vi "SVPWMTimingAlphaBetaFXP_src.vi"(0 "alpha":fxp<+/-,32,4> caption="voltage alpha", 1 "max":fxp<+/-,32,4>=0.999969482421875 caption="max voltage", 2 "Period":u32, 5 "beta":fxp<+/-,32,4> caption="voltage beta") -> (4 "U_Timing":T1, 6 "V_Timing":T1, 8 "W_timing":T1, 15 "Sector":u8)   [LabVIEW 2015]
uses:
  ON_OFF_timing.ctl
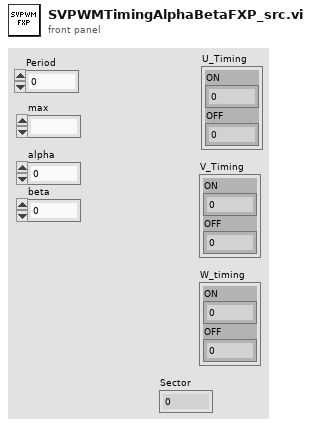
[diagram p1: front panel]
types:
  T1 = typedef "ON_OFF_timing.ctl" = cluster{"ON":u32, "OFF":u32}
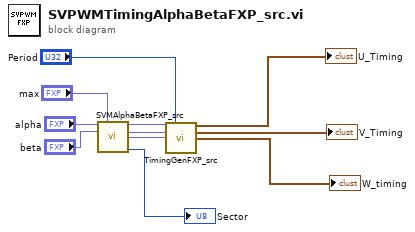
[diagram p0: block diagram]
diagram:
  n1 = call "SVMAlphaBetaFXP_src.vi"("alpha"="alpha", "max"="max", "beta"="beta") -> ("Upercent"=w11:fxp<+/-,32,4>, "Vpercent"=w10:fxp<+/-,32,4>, "Wpercent"=w9:fxp<+/-,32,4>, "Sector"=→"Sector":u8)  [unwired: 9 in]
  n2 = call "TimingGenFXP_src.vi"("Upercent"=w11, "Period"="Period", "Vpercent"=w10, "Wpercent"=w9) -> ("U_Timing"=→"U_Timing":T1, "V_Timing"=→"V_Timing":T1, "W_timing"=→"W_timing":T1)  [unwired: 9 in]
